vi "输入输出模块.vi"(2 "显示内容簇":T2, 3 "方法选择簇":T1) -> (0 "显示项":T2)   [LabVIEW 2018]
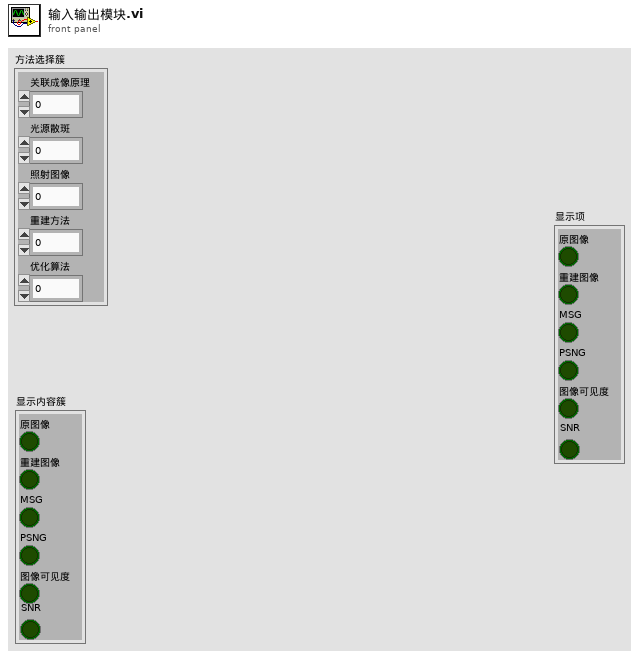
[diagram p1: front panel]
types:
  T1 = cluster{"关联成像原理":i32, "光源散斑":i32, "照射图像":i32, "重建方法":i32, "优化算法":i32}
  T2 = cluster{"原图像":bool, "重建图像":bool, "MSG":bool, "PSNG":bool, "图像可见度":bool, "SNR":bool}
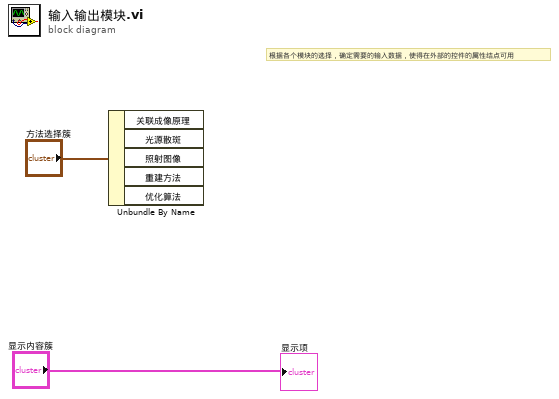
[diagram p0: block diagram]
diagram:
  # "根据各个模块的选择，确定需要的输入数据，使得在外部的控件的属性结点可用"
  n1 = Unbundle By Name("方法选择簇") -> ()  [unwired: 5 out]
  "显示项" <- "显示内容簇"
